vi "SimulatedCreateChannel.vi"(8 "error in (no error)":errorcluster, 9 "Unit":string, 10 "Name":string, 11 "HardwareChannel":string) -> (0 "error out":errorcluster)   [LabVIEW 2017, in "EmsaAcquisition.lvlib"]
uses:
  <vilib>/addons/InsightCM/Devices/Shared/Emsa/EmsaAcquisition/EmsaAcquisition.lvlib
  <vilib>/addons/InsightCM/Devices/Shared/Emsa/EmsaAcquisition/subVIs/SimulatedConfigRefGlobal.vi
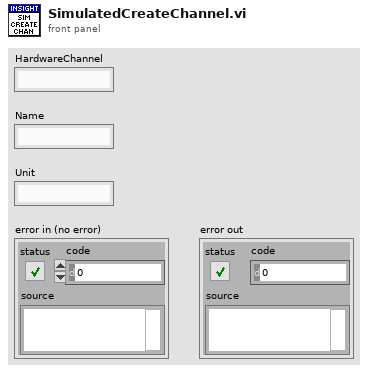
[diagram p1: front panel]
types:
  T1 = typedef "EmsaAcquisition.lvlib/SimulatedConfigRefs.ctl" = cluster{"SimulatedSignalConfig":refnum<vi>}
  T2 = typedef "EmsaAcquisition.lvlib/SimulatedSignalConfig.ctl" = cluster{"Channel Name":string[], "Valid":bool[], "Hardware Channel":string[], "Unit":string[], "Sweep Configs":T3[]}
  T3 = typedef "EmsaAcquisition.lvlib/SimulatedSweepConfig.ctl" = cluster{"Sweep Frequency List":cluster{"frequency":dbl, "bandwidth":dbl}[], "Detection Time":dbl, "Detection Mode":enum16{"Peak", "Quasi Peak", "Average"}, "Full Scale Volts":dbl, "Total Sweep Pts":i32, "Sweep Pointer":i32, "Sweep":T4[], "Sweep Start Time":timestamp}
  T4 = typedef "EmsaAcquisition.lvlib/SweepElement.ctl" = cluster{"Frequency":dbl, "Amplitude":dbl}
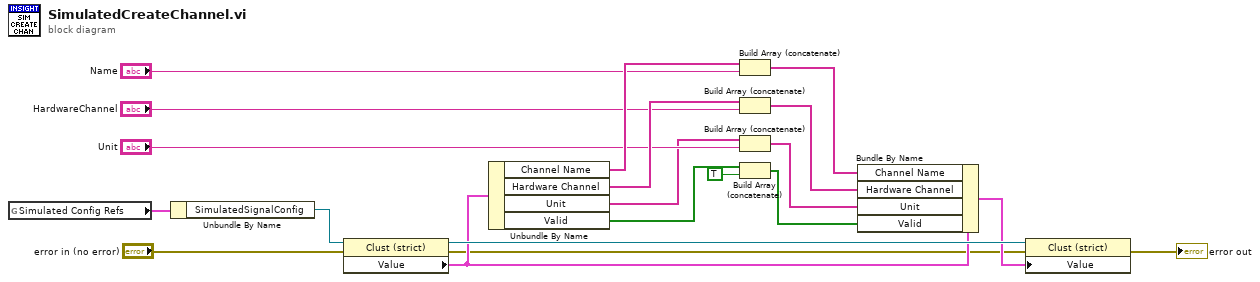
[diagram p0: block diagram]
diagram:
  n1 = global read "SimulatedConfigRefGlobal.vi" "Simulated Config Refs"() -> (w20:T1)
  n2 = Unbundle By Name(w20) -> ("SimulatedSignalConfig"=w19:refnum<vi>)
  n3 = property class="Clust (strict)"(reference=w19, error in="error in (no error)") -> (reference out=w9:refnum<vi>, error out=w1:errorcluster, "Value"=w7:T2)
  n4 = Unbundle By Name(w7) -> ("Channel Name"=w17:string[], "Hardware Channel"=w15:string[], "Unit"=w12:string[], "Valid"=w11:bool[])
  n5 = Build Array (concatenate)(w17, "Name") -> (w3:string[])
  n6 = Build Array (concatenate)(w15, "HardwareChannel") -> (w4:string[])
  n7 = Build Array (concatenate)(w12, "Unit") -> (w5:string[])
  n8 = Build Array (concatenate)(w11, TRUE ("Boolean 2")) -> (w6:bool[])
  n9 = Bundle By Name(cluster=w7, "Channel Name"=w3, "Hardware Channel"=w4, "Unit"=w5, "Valid"=w6) -> (w2:T2)
  n10 = property class="Clust (strict)"(reference=w9, error in=w1, "Value"=w2) -> (error out=→"error out":errorcluster)  [unwired: 1 out]
